vi "Stop.vi"(8 "Error In":errorcluster, 11 "reference in":refnum<class "Instrument.lvclass">) -> (0 "Error Out":errorcluster, 3 "reference out":refnum<class "Instrument.lvclass">)   [LabVIEW 2024, in "HAL.lvlib" / "Instrument.lvclass"]
uses:
  Instrument.lvclass
  Configurations/CFG Base/CFG Base.lvclass
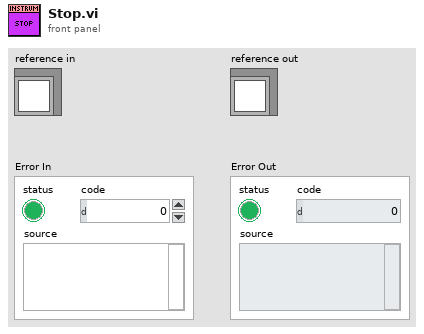
[diagram p1: front panel]
types:
  T1 = typedef "HAL.lvlib/Instrument.lvclass/ObjectAttributes.ctl" = cluster{"CFG Base":refnum<class "CFG Base.lvclass">, "Started Counter":i16}
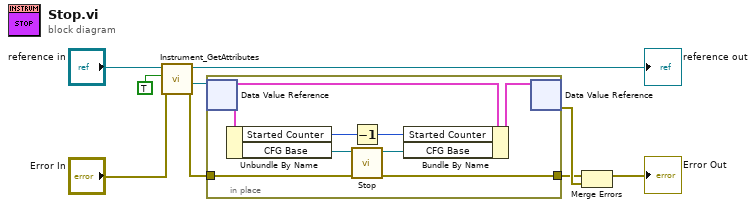
[diagram p0: block diagram]
diagram:
  n1 = call "Instrument_GetAttributes.vi"("Error In"="Error In", "OnlyGetDvrReference(False)"=TRUE, "reference in"="reference in") -> ("Error Out"=w2:errorcluster, "DataRef"=w4:refnum<data-value>, "reference out"=→"reference out":refnum<class "Instrument.lvclass">)  [unwired: 5 in, 1 out]
  n2 = in-place {
    in-place-border: w2 -> [w13]
    in-place-border: [w12] -> w1
    n3 = in-place-dvr #1(w4) -> (w16:T1)  [unwired: 1 out]
    n4 = Unbundle By Name(w16) -> ("Started Counter"=w11:i16, "CFG Base"=w14:refnum<class "CFG Base.lvclass">)
    n5 = Decrement(x=w11) -> (x-1=w10:i16)
    n6 = call-dynamic "Stop.vi"("error in"=w13, "CFG Base in"=w14) -> ("error out"=w12:errorcluster, "CFG Base out"=w15:refnum<class "CFG Base.lvclass">)  [unwired: 8 in]
    n7 = Bundle By Name(cluster=w16, "Started Counter"=w10, "CFG Base"=w15) -> (w17:T1)
    n8 = in-place-dvr #1(w17) -> (w5:errorcluster)  [unwired: 1 out]
  }
  n9 = Merge Errors(w1, w5) -> (→"Error Out":errorcluster)
